vi "Read Description.vi"(11 "Dark Roast in":refnum<class "Dark Roast.lvclass">) -> (2 "Description":string)   [LabVIEW 2013, in "Dark Roast.lvclass"]
uses:
  Dark Roast.lvclass
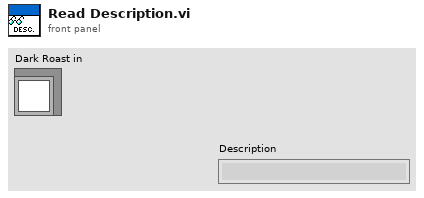
[diagram p1: front panel]
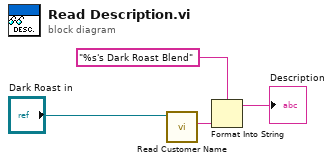
[diagram p0: block diagram]
diagram:
  n1 = call-dynamic "Read Customer Name.vi"("Beverage in"="Dark Roast in") -> ("Customer Name"=w3:string)  [unwired: 10 in]
  n2 = Format Into String(format string="%s's Dark Roast Blend" ("Description"), w3) -> (resulting string=→"Description":string)  [unwired: 2 in, 1 out]
